vi "Inventory-TreeRefs.vi"(0 "ERP-Inventory in":refnum<class "ERP-Inventory.lvclass">, 1 "Tree - Stock Inventory":refnum<vi>, 2 "error in (no error)":errorcluster, 5 "Tree - Pull From Iventory":refnum<vi>) -> (6 "ERP-Inventory out":refnum<class "ERP-Inventory.lvclass">, 7 "error out":errorcluster)   [LabVIEW 2013, in "ERP-Inventory.lvclass"]
uses:
  ERP-Inventory.lvclass
  ERP-Inventory.lvclass/ERP-Inventory.ctl
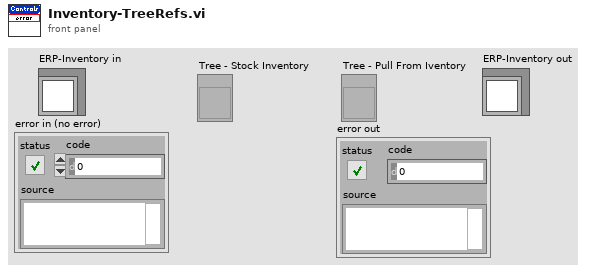
[diagram p1: front panel]
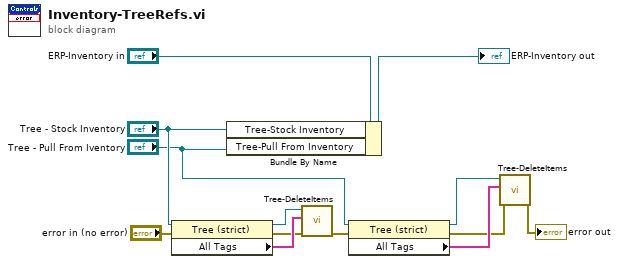
[diagram p0: block diagram]
diagram:
  n1 = property class="Tree (strict)"(reference="Tree - Stock Inventory", error in="error in (no error)") -> (reference out=w9:refnum<vi>, error out=w8:errorcluster, "All Tags"=w10:string[])
  n2 = Bundle By Name(cluster="ERP-Inventory in", "Tree-Stock Inventory"="Tree - Stock Inventory", "Tree-Pull From Inventory"="Tree - Pull From Iventory") -> (→"ERP-Inventory out":refnum<class "ERP-Inventory.lvclass">)
  n3 = call "Tree-DeleteItems.vi"("error In"=w8, "All Tags"=w10, "Tree In"=w9) -> ("error out"=w6:errorcluster)  [unwired: 7 in, 1 out]
  n4 = property class="Tree (strict)"(reference="Tree - Pull From Iventory", error in=w6) -> (reference out=w2:refnum<vi>, error out=w4:errorcluster, "All Tags"=w5:string[])
  n5 = call "Tree-DeleteItems.vi"("error In"=w4, "All Tags"=w5, "Tree In"=w2) -> ("error out"=→"error out":errorcluster)  [unwired: 7 in, 1 out]
